vi "FTW-Time-Timer.vi"(0 "Initial Tick Count":u32 format="%06dmsec", 11 "error in":errorcluster) -> (4 "Current Tick Count":u32 format="%06dmsec", 6 "Elapsed Time":u32 format="%06dmsec", 15 "error out":errorcluster)   [LabVIEW 2012]
panel:
  # "Inputs"
  # "Outputs"
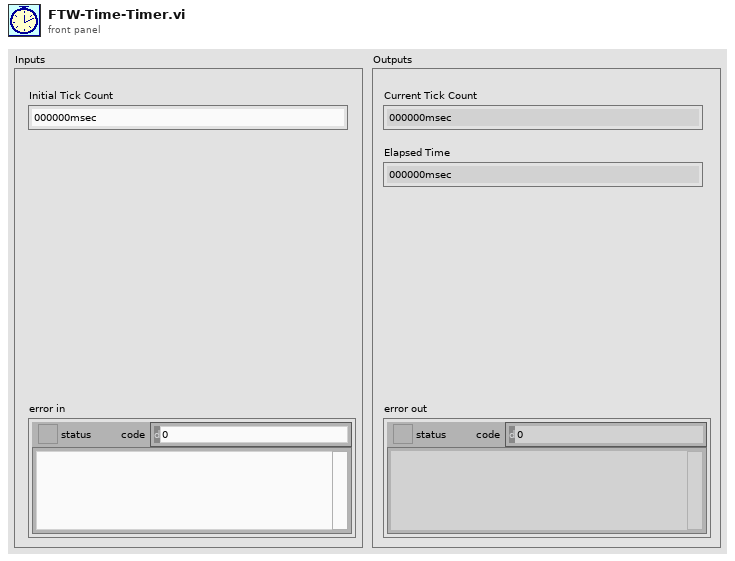
[diagram p1: front panel]
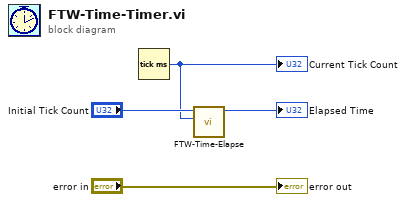
[diagram p0: block diagram]
diagram:
  n1 = Tick Count (ms)() -> (millisecond timer value=w3:u32)
  "Current Tick Count" <- w3
  n2 = call "FTW-Time-Elapse.vi"("End Time"=w3, "Initial Time"="Initial Tick Count") -> ("Elapsed msec"=→"Elapsed Time":u32)  [unwired: 8 in, 1 out]
  "error out" <- "error in"
